vi "MainDataStructure.vi"() -> (0 "Data Structure":T3={"Error"={"status"=FALSE, "code"=0, "source"=""}, "Exit"=FALSE, "All Ref"={"VIRef"=refnum, "CtlRef"=refnum, "界面控件Ref"=refnum}, "System Path"={"Data"=path ""}, "Dynamic VI Path"={"Thread Path"=path ""}, "Reentrant VI Path"={"Reentrant Thread Path"=path "", "Reentrant VI Count"=0}, "Engine Path"={"Engine Path"=path ""}, "Main VI"={"Main Name"="", "Main Order"="", "Main Data"=variant}, "Engine"={"Engine Path"=path "", "Engine Name"="", "Engine Order"="", "Engine Data"=variant}, "Thread to Operate"={"Thread VI Path"=path "", "Invoke Property"={"open front panel? (T)"=FALSE, "Reentrant? (F)"=FALSE, "Insert to Subpanel?(F)"=FALSE, "time out(5s)"=0.0}, "Queue Info"={"HighLevel Thread"="", "Thread Q Name"="", "Data"=variant}}, "Send Data to Thread"={"Thread to Send"=[], "Order to Send"=[], "Data to Send"=[]}, "Dynamic Threads Array"=[], "控件排布前面板"={"获取引用"={"获取VI引用句柄"=refnum, "获取Ctl引用句柄"=refnum}, "位置_前"={"位置"={"Horizontal"=25, "Vertical"=250}}, "创建控件"={"创建数量"=0}, "lNameLable"=[]}, "控件排布后面板"={"位置_后"={"位置"={"Horizontal"=25, "Vertical"=250}}}, "DynamicThreadsPath"={"ReOriginVI"=path ""}, "界面控件"={"当前选择路径"=path "", "控件名称"="", "颜色盒"=0, "名称列表路径"=path "", "名称列表"=[], "类名"=""}})   [LabVIEW 2018]
uses:
  <vilib>/Utility/miscctls.llb/LVPointTypeDef.ctl
  DynamicThreads.ctl
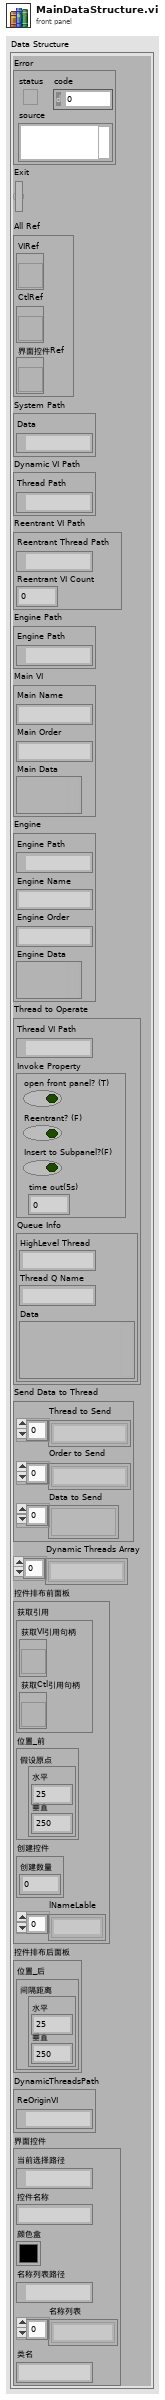
[diagram p1: front panel]
types:
  T1 = typedef "LVPointTypeDef.ctl" = cluster{"Horizontal":i16, "Vertical":i16}
  T2 = typedef "DynamicThreads.ctl" = cluster{"ReOriginVI":path}
  T3 = cluster{"Error":errorcluster, "Exit":bool, "All Ref":cluster{"VIRef":refnum<vi>, "CtlRef":refnum<vi>, "界面控件Ref":refnum<vi>}, "System Path":cluster{"Data":path}, "Dynamic VI Path":cluster{"Thread Path":path}, "Reentrant VI Path":cluster{"Reentrant Thread Path":path, "Reentrant VI Count":u32}, "Engine Path":cluster{"Engine Path":path}, "Main VI":cluster{"Main Name":string, "Main Order":string, "Main Data":variant}, "Engine":cluster{"Engine Path":path, "Engine Name":string, "Engine Order":string, "Engine Data":variant}, "Thread to Operate":cluster{"Thread VI Path":path, "Invoke Property":cluster{"open front panel? (T)":bool, "Reentrant? (F)":bool, "Insert to Subpanel?(F)":bool, "time out(5s)":dbl}, "Queue Info":cluster{"HighLevel Thread":string, "Thread Q Name":string, "Data":variant}}, "Send Data to Thread":cluster{"Thread to Send":string[], "Order to Send":string[], "Data to Send":variant[]}, "Dynamic Threads Array":string[], "控件排布前面板":cluster{"获取引用":cluster{"获取VI引用句柄":refnum<vi>, "获取Ctl引用句柄":refnum<vi>}, "位置_前":cluster{"位置":T1}, "创建控件":cluster{"创建数量":u16}, "lNameLable":string[]}, "控件排布后面板":cluster{"位置_后":cluster{"位置":T1}}, "DynamicThreadsPath":T2, "界面控件":cluster{"当前选择路径":path, "控件名称":string, "颜色盒":u32, "名称列表路径":path, "名称列表":string[], "类名":string}}
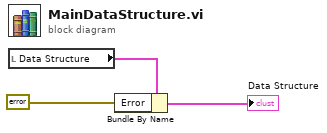
[diagram p0: block diagram]
diagram:
  n1 = local read "Data Structure"() -> (w2:T3)
  n2 = Bundle By Name(cluster=w2, "Error"=errorcluster {"status"=FALSE, "code"=0, "source"=""}) -> (→"Data Structure":T3)
